vi "SetupJog.vi"(8 "error in (no error)":errorcluster, 10 "jogDistance":dbl, 11 "KST101 in":refnum<class "KST101.lvclass">) -> (0 "error out":errorcluster, 3 "KST101 out":refnum<class "KST101.lvclass">)   [LabVIEW 2016, in "Stepper Motor Controller.lvlib" / "KST101.lvclass"]
uses:
  KST101.lvclass
  KST101.lvclass/KST101.ctl
  D:/Workspace/ProCyteOne_LaserModuleAlignment/shared/Thorlabs/Kinesis/Dependencies/Thorlabs.MotionControl.KCube.StepperMotorCLI.dll
  Dependencies/Thorlabs.MotionControl.KCube.StepperMotorCLI.dll
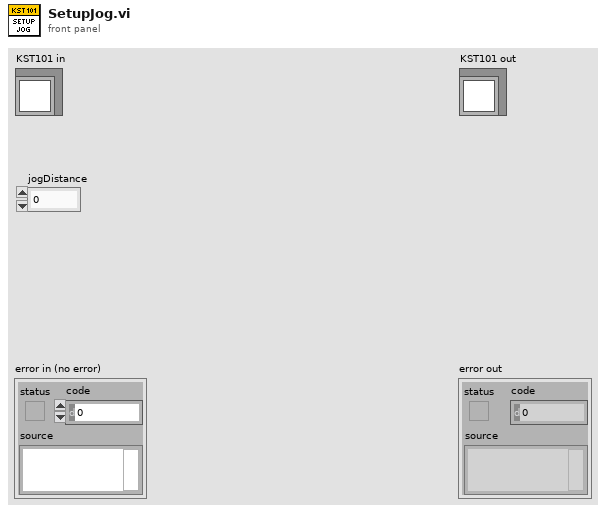
[diagram p1: front panel]
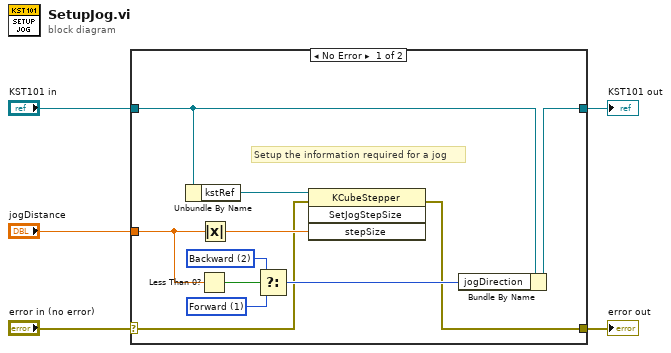
[diagram p0: block diagram]
diagram:
  n1 = case shown="No Error" "error in (no error)" {
    selector: "error in (no error)" -> [w7 w18]
    tunnel: [w6 w18] -> w4
    tunnel: [w11 w17] -> w2
    tunnel: "KST101 in" -> [w12 w17]
    tunnel: "jogDistance" -> [w14 _]
    frame No Error {
      w10 = 2 items=["Forward"=1, "Backward"=2] ("jogDirection")
      w9 = 1 items=["Forward"=1, "Backward"=2] ("jogDirection")
      # "Setup the information required for a jog"
      n2 = Unbundle By Name(w12) -> ("kstRef"=w16:refnum<k24>)
      n3 = Less Than 0?(x=w14) -> (x < 0?=w15:bool)
      n4 = Absolute Value(x=w14) -> (abs(x)=w13:dbl)
      n5 = Select(t=w10, s=w15, f=w9) -> (s? t:f=w8:i32)
      n6 = invoke class="KCubeStepper" method="SetJogStepSize"(reference=w16, error in=w7, "stepSize"=w13) -> (error out=w6:errorcluster)  [unwired: 1 in, 3 out]
      n7 = Bundle By Name(cluster=w12, "jogDirection"=w8) -> (w11:refnum<class "KST101.lvclass">)
    }
    frame Error {
    }
  }
  "error out" <- w4
  "KST101 out" <- w2
